vi "Data_Save_MAX.vi"(9 "Data":T1) -> (2 "max":string[](array[string]))   [LabVIEW 2017]
uses:
  Ctrls/Data.ctl
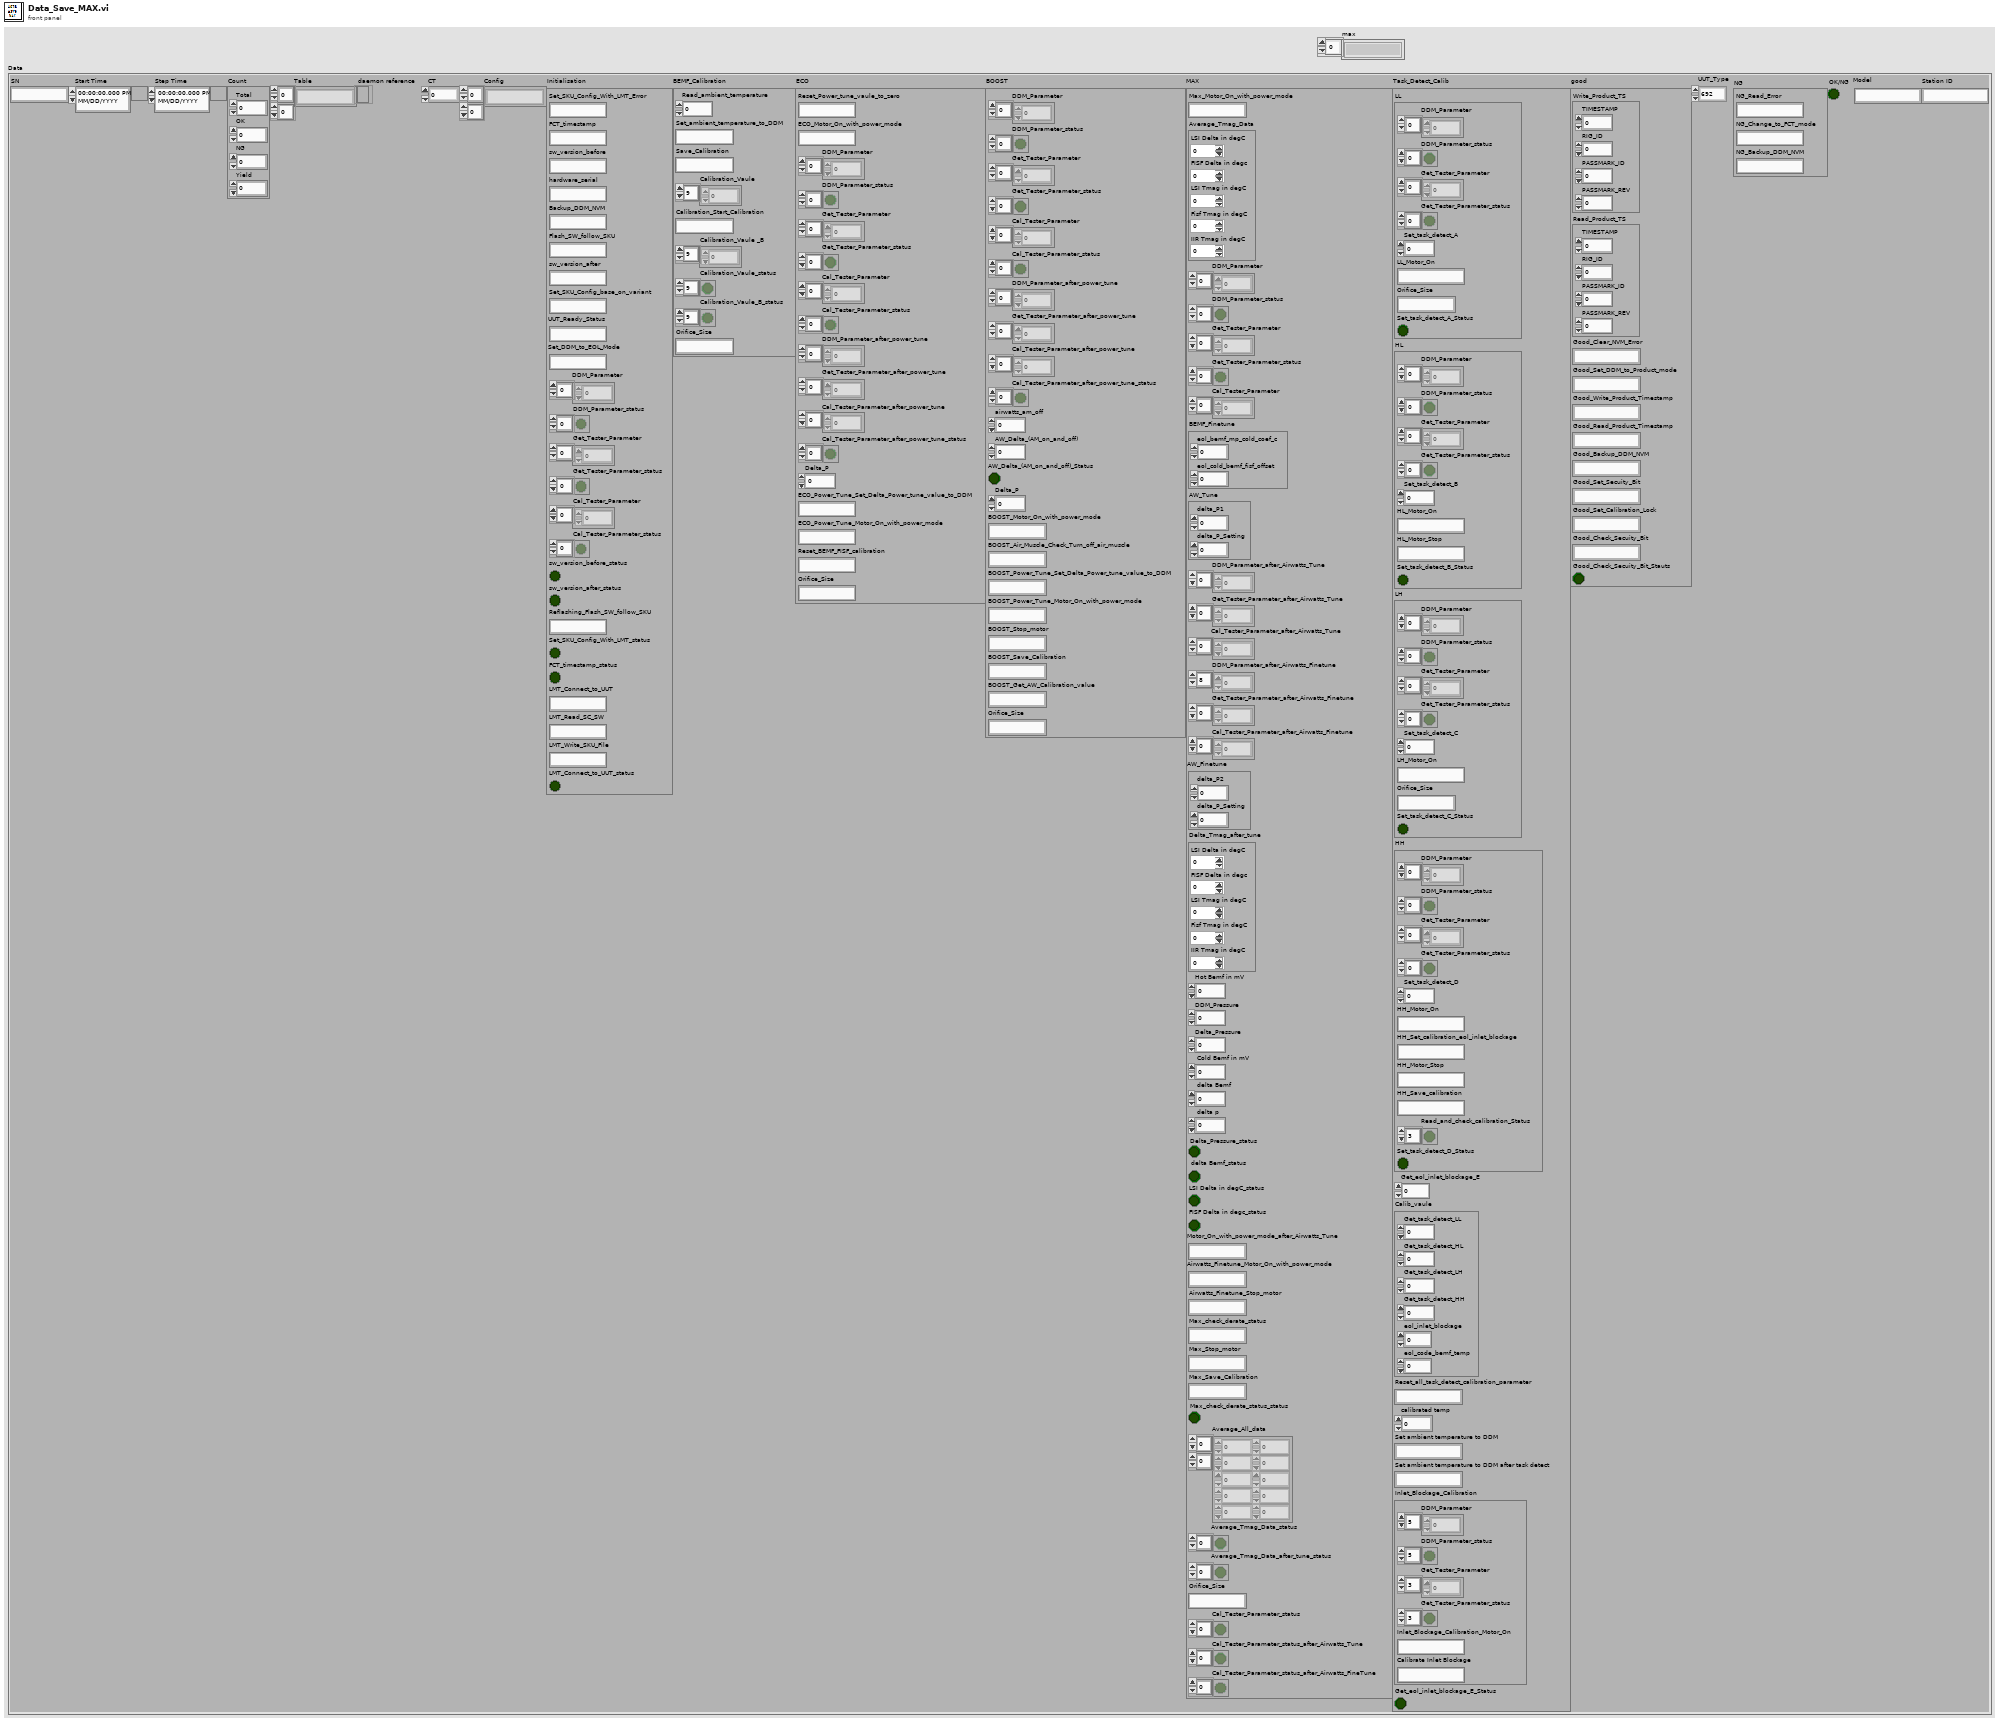
[diagram p1: front panel]
types:
  T1 = typedef "Data.ctl" = cluster{"SN":string, "Start Time":timestamp, "Step Time":timestamp, "Count":cluster{"Total":i32, "OK":i32, "NG":i32, "Yield":dbl}, "Table":string[][], "daemon reference":refnum<k5>, "CT":dbl, "Config":string[][], "Initialisation":cluster{"Set_SKU_Config_With_LMT_Error":string, "FCT_timestamp":string, "sw_version_before":string, "hardware_serial":string, "Backup_DDM_NVM":string, "Flash_SW_follow_SKU":string, "sw_version_after":string, "Set_SKU_Config_base_on_variant":string, "UUT_Ready_Status":string, "Set_DDM_to_EOL_Mode":string, "DDM_Parameter":dbl[], "DDM_Parameter_status":bool[], "Get_Tester_Parameter":dbl[], "Get_Tester_Parameter_status":bool[], "Cal_Tester_Parameter":dbl[], "Cal_Tester_Parameter_status":bool[], "sw_version_before_status":bool, "sw_version_after_status":bool, "Reflashing_Flash_SW_follow_SKU":string, "Set_SKU_Config_With_LMT_status":bool, "FCT_timestamp_status":bool, "LMT_Connect_to_UUT":string, "LMT_Read_SC_SW":string, "LMT_Write_SKU_File":string, "LMT_Connect_to_UUT_status":bool}, "BEMF_Calibration":cluster{"Read_ambient_temperature":dbl, "Set_ambient_temperature_to_DDM":string, "Save_Calibration":string, "Calibration_Vaule":dbl[], "Calibration_Start_Calibration":string, "Calibration_Vaule _B":dbl[], "Calibration_Vaule_status":bool[], "Calibration_Vaule_B_status":bool[], "Orifice_Size":string}, "ECO":cluster{"Reset_Power_tune_vaule_to_zero":string, "ECO_Motor_On_with_power_mode":string, "DDM_Parameter":dbl[], "DDM_Parameter_status":bool[], "Get_Tester_Parameter":dbl[], "Get_Tester_Parameter_status":bool[], "Cal_Tester_Parameter":dbl[], "Cal_Tester_Parameter_status":bool[], "DDM_Parameter_after_power_tune":dbl[], "Get_Tester_Parameter_after_power_tune":dbl[], "Cal_Tester_Parameter_after_power_tune":dbl[], "Cal_Tester_Parameter_after_power_tune_status":bool[], "Delta_P":dbl, "ECO_Power_Tune_Set_Delta_Power_tune_value_to_DDM":string, "ECO_Power_Tune_Motor_On_with_power_mode":string, "Reset_BEMF_FISF_calibration":string, "Orifice_Size":string}, "BOOST":cluster{"DDM_Parameter":dbl[], "DDM_Parameter_status":bool[], "Get_Tester_Parameter":dbl[], "Get_Tester_Parameter_status":bool[], "Cal_Tester_Parameter":dbl[], "Cal_Tester_Parameter_status":bool[], "DDM_Parameter_after_power_tune":dbl[], "Get_Tester_Parameter_after_power_tune":dbl[], "Cal_Tester_Parameter_after_power_tune":dbl[], "Cal_Tester_Parameter_after_power_tune_status":bool[], "airwatts_am_off":dbl, "AW_Delta_(AM_on_and_off)":dbl, "AW_Delta_(AM_on_and_off)_Status":bool, "Delta_P":dbl, "BOOST_Motor_On_with_power_mode":string, "BOOST_Air_Muscle_Check_Turn_off_air_muscle":string, "BOOST_Power_Tune_Set_Delta_Power_tune_value_to_DDM":string, "BOOST_Power_Tune_Motor_On_with_power_mode":string, "BOOST_Stop_motor":string, "BOOST_Save_Calibration":string, "BOOST_Get_AW_Calibration_value":string, "Orifice_Size":string}, "MAX":cluster{"Max_Motor_On_with_power_mode":string, "Average_Tmag_Data":cluster{"LSI Delta in degC":dbl, "FISF Delta in degc":dbl, "LSI Tmag in degC":dbl, "Fisf Tmag in degC":dbl, "IIR Tmag in degC":dbl}, "DDM_Parameter":dbl[], "DDM_Parameter_status":bool[], "Get_Tester_Parameter":dbl[], "Get_Tester_Parameter_status":bool[], "Cal_Tester_Parameter":dbl[], "BEMF_Finetune":cluster{"eol_bemf_mp_cold_coef_c":dbl, "eol_cold_bemf_fisf_offset":dbl}, "AW_Tune":cluster{"delta_P1":dbl, "delta_P_Setting":dbl}, "DDM_Parameter_after_Airwatts_Tune":dbl[], "Get_Tester_Parameter_after_Airwatts_Tune":dbl[], "Cal_Tester_Parameter_after_Airwatts_Tune":dbl[], "DDM_Parameter_after_Airwatts_Finetune":dbl[], "Get_Tester_Parameter_after_Airwatts_Finetune":dbl[], "Cal_Tester_Parameter_after_Airwatts_Finetune":dbl[], "AW_Finetune":cluster{"delta_P2":dbl, "delta_P_Setting":dbl}, "Delta_Tmag_after_tune":cluster{"LSI Delta in degC":dbl, "FISF Delta in degc":dbl, "LSI Tmag in degC":dbl, "Fisf Tmag in degC":dbl, "IIR Tmag in degC":dbl}, "Hot Bemf in mV":dbl, "DDM_Pressure":dbl, "Delta_Pressure":dbl, " Cold Bemf in mV":dbl, " delta Bemf":dbl, " delta p":dbl, "Delta_Pressure_status":bool, " delta Bemf_status":bool, "LSI Delta in degC_status":bool, "FISF Delta in degc_status":bool, "Motor_On_with_power_mode_after_Airwatts_Tune":string, "Airwatts_Finetune_Motor_On_with_power_mode":string, "Airwatts_Finetune_Stop_motor":string, "Max_check_derate_status":string, "Max_Stop_motor":string, "Max_Save_Calibration":string, "Max_check_derate_status_status":bool, "Average_All_data":dbl[][], "Average_Tmag_Data_status":bool[], "Average_Tmag_Data_after_tune_status":bool[], "Orifice_Size":string, "Cal_Tester_Parameter_status":bool[], "Cal_Tester_Parameter_status_after_Airwatts_Tune":bool[], "Cal_Tester_Parameter_status_after_Airwatts_FineTune":bool[]}, "Task_Detect_Calib":cluster{"LL":cluster{"DDM_Parameter":dbl[], "DDM_Parameter_status":bool[], "Get_Tester_Parameter":dbl[], "Get_Tester_Parameter_status":bool[], "Set_task_detect_A":dbl, "LL_Motor_On":string, "Orifice_Size":string, "Set_task_detect_A_Status":bool}, "HL":cluster{"DDM_Parameter":dbl[], "DDM_Parameter_status":bool[], "Get_Tester_Parameter":dbl[], "Get_Tester_Parameter_status":bool[], "Set_task_detect_B":dbl, "HL_Motor_On":string, "HL_Motor_Stop":string, "Set_task_detect_B_Status":bool}, "LH":cluster{"DDM_Parameter":dbl[], "DDM_Parameter_status":bool[], "Get_Tester_Parameter":dbl[], "Get_Tester_Parameter_status":bool[], "Set_task_detect_C":dbl, "LH_Motor_On":string, "Orifice_Size":string, "Set_task_detect_C_Status":bool}, "HH":cluster{"DDM_Parameter":dbl[], "DDM_Parameter_status":bool[], "Get_Tester_Parameter":dbl[], "Get_Tester_Parameter_status":bool[], "Set_task_detect_D":dbl, "HH_Motor_On":string, "HH_Set_calibration_eol_inlet_blockage":string, "HH_Motor_Stop":string, "HH_Save_calibration":string, "Read_and_check_calibration_Status":bool[], "Set_task_detect_D_Status":bool}, "Get_eol_inlet_blockage_E":dbl, "Calib_vaule":cluster{"Get_task_detect_LL":dbl, "Get_task_detect_HL":dbl, "Get_task_detect_LH":dbl, "Get_task_detect_HH":dbl, "eol_inlet_blockage":dbl, "eol_code_bemf_temp":dbl}, "Reset_all_task_detect_calibration_parameter":string, "calibrated temp":dbl, "Set ambient temperature to DDM":string, "Set ambient temperature to DDM after task detect":string, "Inlet_Blockage_Calibration":cluster{"DDM_Parameter":dbl[], "DDM_Parameter_status":bool[], "Get_Tester_Parameter":dbl[], "Get_Tester_Parameter_status":bool[], "Inlet_Blockage_Calibration_Motor_On":string, "Calibrate Inlet Blockage":string}, "Get_eol_inlet_blockage_E_Status":bool}, "good":cluster{"Write_Product_TS":cluster{"TIMESTAMP":i64, "RIG_ID":i64, "PASSMARK_ID":i64, "PASSMARK_REV":i64}, "Read_Product_TS":cluster{"TIMESTAMP":i64, "RIG_ID":i64, "PASSMARK_ID":i64, "PASSMARK_REV":i64}, "Good_Clear_NVM_Error":string, "Good_Set_DDM_to_Product_mode":string, "Good_Write_Product_Timestamp":string, "Good_Read_Product_Timestamp":string, "Good_Backup_DDM_NVM":string, "Good_Set_Secuity_Bit":string, "Good_Set_Calibration_Lock":string, "Good_Check_Secuity_Bit":string, "Good_Check_Secuity_Bit_Stauts":bool}, "UUT_Type":enum16{"692", "692B", "692D"}, "NG":cluster{"NG_Read_Error":string, "NG_Change_to_FCT_mode":string, "NG_Backup_DDM_NVM":string}, "OK/NG":bool, "Model":string, "Station ID":string}
  T2 = cluster{"LSI Delta in degC":dbl, "FISF Delta in degc":dbl, "LSI Tmag in degC":dbl, "Fisf Tmag in degC":dbl, "IIR Tmag in degC":dbl}
  T3 = typedef "HD Config.ctl" = cluster{" PC":cluster{"PC Address":u8[], "PC Port":i32}, "FCO":cluster{"COM":refnum<visa-resource-name>, "Baudrate":u32}, "DC Power ":cluster{"COM":refnum<visa-resource-name>, "Baudrate":u32}, "PW3336":cluster{"COM":refnum<visa-resource-name>, "Baudrate":u32}, "Lefoo":cluster{"COM":refnum<visa-resource-name>, "Baudrate":u32}, "AI Model":cluster{"COM":refnum<visa-resource-name>, "Baudrate":u32}, "DIPC":cluster{"COM":refnum<visa-resource-name>}, "Daemon":cluster{"IP Address":string, "Port":u16, "Retry":u16}, "Motor":cluster{"COM":refnum<visa-resource-name>, "Baudrate":u32}, "G1":bool, "Fail_resume_mode":bool, "Skip DDM Speed&Pressure Passmark":bool}
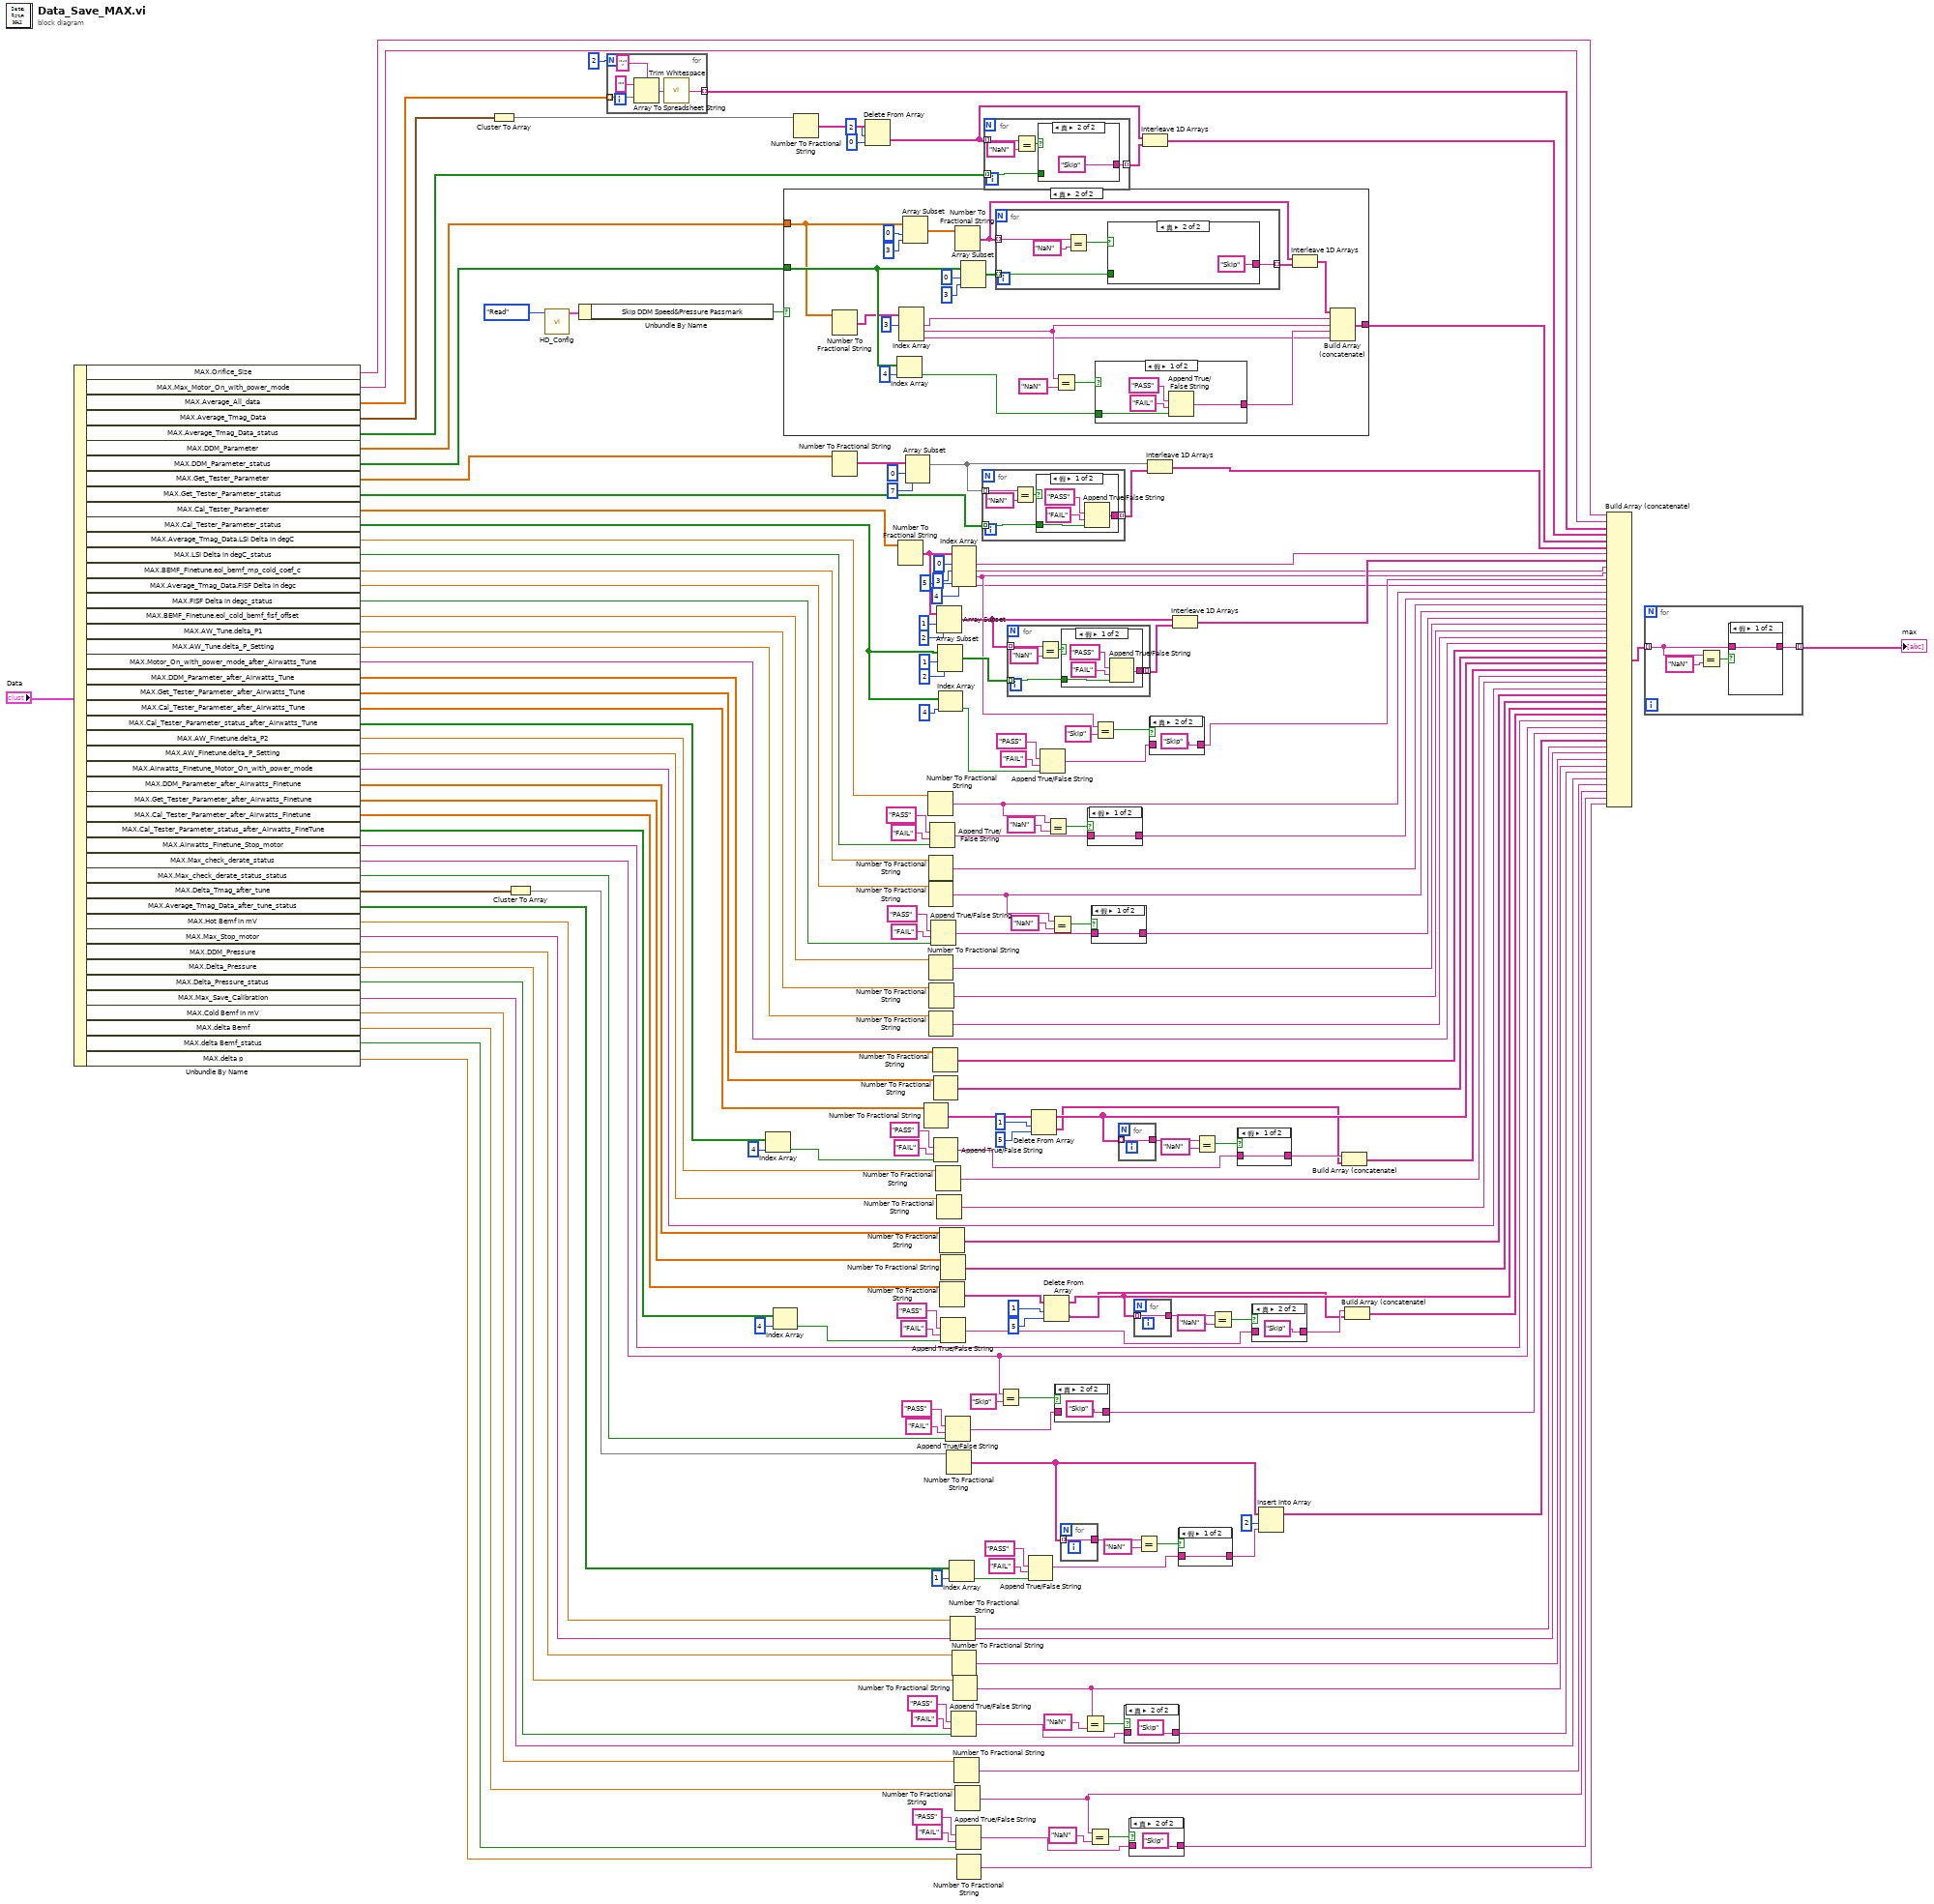
[diagram p0: block diagram]
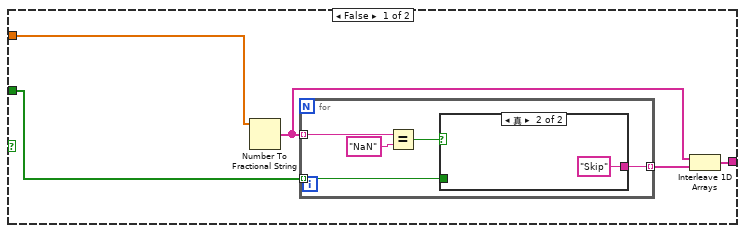
[diagram p2: hidden frame]
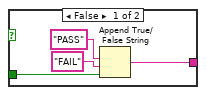
[diagram p3: hidden frame]
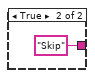
[diagram p4: hidden frame]
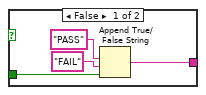
[diagram p5: hidden frame]
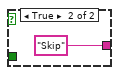
[diagram p7: hidden frame]
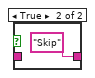
[diagram p8: hidden frame]
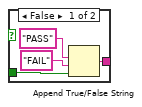
[diagram p9: hidden frame]
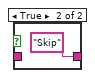
[diagram p14: hidden frame]
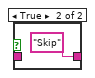
[diagram p15: hidden frame]
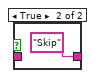
[diagram p16: hidden frame]
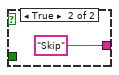
[diagram p17: hidden frame]
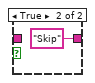
[diagram p18: hidden frame]
diagram:
  n1 = Unbundle By Name("Data") -> ("MAX.Orifice_Size"=w56:string, "MAX.Max_Motor_On_with_power_mode"=w57:string, "MAX.Average_All_data"=w80:dbl[][], "MAX.Average_Tmag_Data"=w177:T2, "MAX.Average_Tmag_Data_status"=w75:bool[], "MAX.DDM_Parameter"=w24:dbl[], "MAX.DDM_Parameter_status"=w23:bool[], "MAX.Get_Tester_Parameter"=w175:dbl[], "MAX.Get_Tester_Parameter_status"=w126:bool[], "MAX.Cal_Tester_Parameter"=w174:dbl[], "MAX.Cal_Tester_Parameter_status"=w47:bool[], "MAX.Average_Tmag_Data.LSI Delta in degC"=w172:dbl, "MAX.LSI Delta in degC_status"=w171:bool, "MAX.BEMF_Finetune.eol_bemf_mp_cold_coef_c"=w170:dbl, "MAX.Average_Tmag_Data.FISF Delta in degc"=w169:dbl, "MAX.FISF Delta in degc_status"=w168:bool, "MAX.BEMF_Finetune.eol_cold_bemf_fisf_offset"=w167:dbl, "MAX.AW_Tune.delta_P1"=w166:dbl, "MAX.AW_Tune.delta_P_Setting"=w165:dbl, "MAX.Motor_On_with_power_mode_after_Airwatts_Tune"=w160:string, "MAX.DDM_Parameter_after_Airwatts_Tune"=w159:dbl[], "MAX.Get_Tester_Parameter_after_Airwatts_Tune"=w158:dbl[], "MAX.Cal_Tester_Parameter_after_Airwatts_Tune"=w14:dbl[], "MAX.Cal_Tester_Parameter_status_after_Airwatts_Tune"=w155:bool[], "MAX.AW_Finetune.delta_P2"=w154:dbl, "MAX.AW_Finetune.delta_P_Setting"=w153:dbl, "MAX.Airwatts_Finetune_Motor_On_with_power_mode"=w150:string, "MAX.DDM_Parameter_after_Airwatts_Finetune"=w147:dbl[], "MAX.Get_Tester_Parameter_after_Airwatts_Finetune"=w146:dbl[], "MAX.Cal_Tester_Parameter_after_Airwatts_Finetune"=w145:dbl[], "MAX.Cal_Tester_Parameter_status_after_Airwatts_FineTune"=w144:bool[], "MAX.Airwatts_Finetune_Stop_motor"=w141:string, "MAX.Max_check_derate_status"=w84:string, "MAX.Max_check_derate_status_status"=w86:bool, "MAX.Delta_Tmag_after_tune"=w176:T2, "MAX.Average_Tmag_Data_after_tune_status"=w71:bool[], "MAX.Hot Bemf in mV"=w139:dbl, "MAX.Max_Stop_motor"=w137:string, "MAX.DDM_Pressure"=w136:dbl, "MAX.Delta_Pressure"=w89:dbl, "MAX.Delta_Pressure_status"=w92:bool, "MAX.Max_Save_Calibration"=w134:string, "MAX.Cold Bemf in mV"=w133:dbl, "MAX.delta Bemf"=w132:dbl, "MAX.delta Bemf_status"=w100:bool, "MAX.delta p"=w131:dbl)
  n2 = Cluster To Array(cluster=w177) -> (array=w173:dbl[])
  n3 = Cluster To Array(cluster=w176) -> (array=w140:dbl[])
  n4 = call "HD_Config.vi"("Step"=enum16{"Initial", "Write", "Read"}."Read") -> ("HD Config out"=w26:T3)  [unwired: 9 in, 1 out]
  n5 = Unbundle By Name(w26) -> ("Skip DDM Speed&Pressure Passmark"=w25:bool)
  n6 = for {
    N: 2 -> [_]
    tunnel: w80 -> [w189] mode=indexing
    tunnel: [w185] -> w79 mode=indexing
    n7 = Array To Spreadsheet String(delimiter (Tab)=";", array=w189, 3:"" ("format string")) -> (spreadsheet string=w186:string)
    n8 = call <vilib>:"Trim Whitespace.vi"("string"=w186) -> ("trimmed string"=w185:string)  [unwired: 1 in]
  }
  n9 = Index Array(array=w155, index=4) -> (element=w34:bool)
  n10 = Index Array(array=w144, index=4) -> (element=w32:bool)
  n11 = case shown="真" w25 {
    tunnel: w23 -> [w190 w216]
    tunnel: w24 -> [w191 w213]
    tunnel: [w192 w205] -> w22
    frame False {
      n12 = Number To Fractional String(number=w191) -> (F-format string=w193:string[])  [unwired: 3 in]
      n13 = for {
        tunnel: w190 -> [w199] mode=indexing
        tunnel: [w198] -> w194 mode=indexing
        tunnel: w193 -> [w196] mode=indexing
        n14 = Equal?(x=w196, y="NaN" ("x")) -> (x = y?=w195:bool)
        n15 = case shown="真" w195 {
          tunnel: w199 -> [w203 _]
          tunnel: [w201 "Skip" ("x")] -> w198
          frame False {
            n16 = Append True/False String(1:w203, 2:"FAIL" ("字符串(\"\")"), 3:"PASS" ("真字符串")) -> (0:w201:string)  [unwired: 1 in]
          }
          frame True {
          }
        }
      }
      n17 = Interleave 1D Arrays(w193, w194) -> (w192:string[])
    }
    frame True {
      n18 = Number To Fractional String(number=w213) -> (F-format string=w212:string[])  [unwired: 3 in]
      n19 = Index Array(array=w216, index=4 ("索引")) -> (element=w211:bool)
      n20 = Index Array(array=w212, index #1=3 ("索引")) -> (element #1=w210:string, element #2=w208:string, element #3=w207:string)  [unwired: 2 in]
      n21 = Array Subset(array=w213, index=0 ("索引"), length=3 ("长度")) -> (w224:dbl[])
      n22 = Number To Fractional String(number=w224) -> (F-format string=w219:string[])  [unwired: 3 in]
      n23 = Array Subset(array=w216, index=0 ("索引"), length=3 ("长度")) -> (w225:bool[])
      n24 = for {
        tunnel: w225 -> [w236] mode=indexing
        tunnel: [w235] -> w226 mode=indexing
        tunnel: w219 -> [w233] mode=indexing
        n25 = Equal?(x=w233, y="NaN" ("x")) -> (x = y?=w232:bool)
        n26 = case shown="真" w232 {
          tunnel: w236 -> [w240 _]
          tunnel: [w238 "Skip" ("x")] -> w235
          frame False {
            n27 = Append True/False String(1:w240, 2:"FAIL" ("字符串(\"\")"), 3:"PASS" ("真字符串")) -> (0:w238:string)  [unwired: 1 in]
          }
          frame True {
          }
        }
      }
      n28 = Equal?(x=w208, y="NaN" ("x")) -> (x = y?=w215:bool)
      n29 = case shown="假" w215 {
        tunnel: w211 -> [w230 _]
        tunnel: [w228 "Skip" ("x")] -> w209
        frame False {
          n30 = Append True/False String(1:w230, 2:"FAIL" ("字符串(\"\")"), 3:"PASS" ("真字符串")) -> (0:w228:string)  [unwired: 1 in]
        }
        frame True {
        }
      }
      n31 = Interleave 1D Arrays(w219, w226) -> (w206:string[])
      n32 = Build Array (concatenate)(w206, w210, w208, w209, w207) -> (w205:string[])
    }
  }
  n33 = Number To Fractional String(number=w173) -> (F-format string=w78:string[])  [unwired: 3 in]
  n34 = Number To Fractional String(number=w175) -> (F-format string=w18:string[])  [unwired: 3 in]
  n35 = Delete From Array(array=w78, length=2, index=0) -> (deleted portion=w74:string[])  [unwired: 1 out]
  n36 = Number To Fractional String(number=w174) -> (F-format string=w55:string[])  [unwired: 3 in]
  n37 = Array Subset(array=w18, index=0 ("索引"), length=7 ("长度")) -> (w21:string[])
  n38 = Number To Fractional String(number=w14) -> (F-format string=w10:string[])  [unwired: 3 in]
  n39 = Number To Fractional String(number=w172) -> (F-format string=w122:string)  [unwired: 3 in]
  n40 = Number To Fractional String(number=w170) -> (F-format string=w164:string)  [unwired: 3 in]
  n41 = Number To Fractional String(number=w169) -> (F-format string=w116:string)  [unwired: 3 in]
  n42 = Number To Fractional String(number=w167) -> (F-format string=w163:string)  [unwired: 3 in]
  n43 = Number To Fractional String(number=w165) -> (F-format string=w161:string)  [unwired: 3 in]
  n44 = Number To Fractional String(number=w166) -> (F-format string=w162:string)  [unwired: 3 in]
  n45 = Append True/False String(1:w171, 2:"FAIL" ("字符串(\"\")"), 3:"PASS" ("真字符串")) -> (0:w121:string)  [unwired: 1 in]
  n46 = Append True/False String(1:w168, 2:"FAIL" ("字符串(\"\")"), 3:"PASS" ("真字符串")) -> (0:w117:string)  [unwired: 1 in]
  n47 = Number To Fractional String(number=w159) -> (F-format string=w157:string[])  [unwired: 3 in]
  n48 = Number To Fractional String(number=w158) -> (F-format string=w156:string[])  [unwired: 3 in]
  n49 = Append True/False String(1:w34, 2:"FAIL" ("字符串(\"\")"), 3:"PASS" ("真字符串")) -> (0:w111:string)  [unwired: 1 in]
  n50 = Number To Fractional String(number=w154) -> (F-format string=w152:string)  [unwired: 3 in]
  n51 = Array Subset(array=w55, index=1, length=2) -> (w45:string[])
  n52 = Number To Fractional String(number=w153) -> (F-format string=w151:string)  [unwired: 3 in]
  n53 = Array Subset(array=w47, index=1, length=2) -> (w44:bool[])
  n54 = Index Array(array=w47, index=4) -> (element=w38:bool)
  n55 = Number To Fractional String(number=w147) -> (F-format string=w143:string[])  [unwired: 3 in]
  n56 = Number To Fractional String(number=w145) -> (F-format string=w5:string[])  [unwired: 3 in]
  n57 = Number To Fractional String(number=w146) -> (F-format string=w142:string[])  [unwired: 3 in]
  n58 = Append True/False String(1:w32, 2:"FAIL" ("字符串(\"\")"), 3:"PASS" ("真字符串")) -> (0:w106:string)  [unwired: 1 in]
  n59 = Append True/False String(1:w86, 2:"FAIL" ("字符串(\"\")"), 3:"PASS" ("真字符串")) -> (0:w82:string)  [unwired: 1 in]
  n60 = Number To Fractional String(number=w140) -> (F-format string=w61:string[])  [unwired: 3 in]
  n61 = Index Array(array=w71, index=1) -> (element=w66:bool)
  n62 = Number To Fractional String(number=w139) -> (F-format string=w138:string)  [unwired: 3 in]
  n63 = Append True/False String(1:w92, 2:"FAIL" ("字符串(\"\")"), 3:"PASS" ("真字符串")) -> (0:w97:string)  [unwired: 1 in]
  n64 = Index Array(array=w55, index #1=0 ("index"), index #2=3 ("index"), index #3=4 ("index"), index #4=5 ("索引")) -> (element #1=w35:string, element #2=w29:string, element #3=w28:string, element #4=w15:string)
  n65 = Number To Fractional String(number=w136) -> (F-format string=w135:string)  [unwired: 3 in]
  n66 = Number To Fractional String(number=w89) -> (F-format string=w91:string)  [unwired: 3 in]
  n67 = Number To Fractional String(number=w133) -> (F-format string=w130:string)  [unwired: 3 in]
  n68 = Number To Fractional String(number=w132) -> (F-format string=w101:string)  [unwired: 3 in]
  n69 = Append True/False String(1:w100, 2:"FAIL" ("字符串(\"\")"), 3:"PASS" ("真字符串")) -> (0:w99:string)  [unwired: 1 in]
  n70 = Number To Fractional String(number=w131) -> (F-format string=w129:string)  [unwired: 3 in]
  n71 = for {
    tunnel: w126 -> [w246] mode=indexing
    tunnel: [w245] -> w125 mode=indexing
    tunnel: w21 -> [w243] mode=indexing
    n72 = Equal?(x=w243, y="NaN" ("x")) -> (x = y?=w242:bool)
    n73 = case shown="假" w242 {
      tunnel: w246 -> [w250 _]
      tunnel: [w248 "Skip" ("x")] -> w245
      frame False {
        n74 = Append True/False String(1:w250, 2:"FAIL" ("字符串(\"\")"), 3:"PASS" ("真字符串")) -> (0:w248:string)  [unwired: 1 in]
      }
      frame True {
      }
    }
  }
  n75 = for {
    tunnel: w75 -> [w256] mode=indexing
    tunnel: [w255] -> w73 mode=indexing
    tunnel: w74 -> [w253] mode=indexing
    n76 = Equal?(x=w253, y="NaN" ("x")) -> (x = y?=w252:bool)
    n77 = case shown="真" w252 {
      tunnel: w256 -> [w260 _]
      tunnel: [w258 "Skip" ("x")] -> w255
      frame False {
        n78 = Append True/False String(1:w260, 2:"FAIL" ("字符串(\"\")"), 3:"PASS" ("真字符串")) -> (0:w258:string)  [unwired: 1 in]
      }
      frame True {
      }
    }
  }
  n79 = Equal?(x=w84, y="Skip" ("x")) -> (x = y?=w83:bool)
  n80 = for {
    tunnel: w44 -> [w266] mode=indexing
    tunnel: [w265] -> w46 mode=indexing
    tunnel: w45 -> [w263] mode=indexing
    n81 = Equal?(x=w263, y="NaN" ("x")) -> (x = y?=w262:bool)
    n82 = case shown="假" w262 {
      tunnel: w266 -> [w270 _]
      tunnel: [w268 "Skip" ("x")] -> w265
      frame False {
        n83 = Append True/False String(1:w270, 2:"FAIL" ("字符串(\"\")"), 3:"PASS" ("真字符串")) -> (0:w268:string)  [unwired: 1 in]
      }
      frame True {
      }
    }
  }
  n84 = Append True/False String(1:w66, 2:"FAIL" ("字符串(\"\")"), 3:"PASS" ("真字符串")) -> (0:w62:string)  [unwired: 1 in]
  n85 = Delete From Array(array=w10, length=1 ("长度"), index=5 ("索引")) -> (deleted portion=w8:string[], array with subset deleted=w11:string[])
  n86 = Append True/False String(1:w38, 2:"FAIL" ("字符串(\"\")"), 3:"PASS" ("真字符串")) -> (0:w43:string)  [unwired: 1 in]
  n87 = Delete From Array(array=w5, length=1 ("长度"), index=5 ("索引")) -> (deleted portion=w1:string[], array with subset deleted=w4:string[])
  n88 = Equal?(x=w122, y="NaN" ("x")) -> (x = y?=w123:bool)
  n89 = Equal?(x=w116, y="NaN" ("x")) -> (x = y?=w119:bool)
  n90 = case shown="真" w83 {
    tunnel: [w272 "Skip" ("x")] -> w81
    tunnel: w82 -> [w272 _]
    frame False {
    }
    frame True {
    }
  }
  n91 = for {
    tunnel: w61 -> [w274] mode=indexing
    tunnel: [w274] -> w63
  }
  n92 = Equal?(x=w91, y="NaN" ("x")) -> (x = y?=w93:bool)
  n93 = case shown="假" w123 {
    tunnel: [w275 "Skip" ("x")] -> w120
    tunnel: w121 -> [w275 _]
    frame False {
    }
    frame True {
    }
  }
  n94 = Equal?(x=w101, y="NaN" ("x")) -> (x = y?=w105:bool)
  n95 = case shown="假" w119 {
    tunnel: [w277 "Skip" ("x")] -> w115
    tunnel: w117 -> [w277 _]
    frame False {
    }
    frame True {
    }
  }
  n96 = Equal?(x=w28, y="Skip" ("x")) -> (x = y?=w42:bool)
  n97 = for {
    tunnel: w11 -> [w279] mode=indexing
    tunnel: [w279] -> w114
  }
  n98 = case shown="真" w93 {
    tunnel: [w280 "Skip" ("x")] -> w90
    tunnel: w97 -> [w280 _]
    frame False {
    }
    frame True {
    }
  }
  n99 = case shown="真" w105 {
    tunnel: [w282 "Skip" ("x")] -> w98
    tunnel: w99 -> [w282 _]
    frame False {
    }
    frame True {
    }
  }
  n100 = for {
    tunnel: w4 -> [w284] mode=indexing
    tunnel: [w284] -> w107
  }
  n101 = Equal?(x=w63, y="NaN" ("x")) -> (x = y?=w65:bool)
  n102 = Interleave 1D Arrays(w74, w73) -> (w72:string[])
  n103 = Interleave 1D Arrays(w21, w125) -> (w17:string[])
  n104 = case shown="真" w42 {
    tunnel: [w285 "Skip" ("x")] -> w37
    tunnel: w43 -> [w285 _]
    frame False {
    }
    frame True {
    }
  }
  n105 = Interleave 1D Arrays(w45, w46) -> (w36:string[])
  n106 = case shown="假" w65 {
    tunnel: [w287 "Skip" ("x")] -> w60
    tunnel: w62 -> [w287 _]
    frame False {
    }
    frame True {
    }
  }
  n107 = Equal?(x=w114, y="NaN" ("x")) -> (x = y?=w112:bool)
  n108 = Equal?(x=w107, y="NaN" ("x")) -> (x = y?=w109:bool)
  n109 = case shown="假" w112 {
    tunnel: [w289 "Skip" ("x")] -> w110
    tunnel: w111 -> [w289 _]
    frame False {
    }
    frame True {
    }
  }
  n110 = case shown="真" w109 {
    tunnel: [w291 "Skip" ("x")] -> w3
    tunnel: w106 -> [w291 _]
    frame False {
    }
    frame True {
    }
  }
  n111 = Insert Into Array(array=w61, index=2, new element=w60) -> (w59:string[])
  n112 = Build Array (concatenate)(w110, w8) -> (w9:string[])
  n113 = Build Array (concatenate)(w3, w1) -> (w2:string[])
  n114 = Build Array (concatenate)(w56, w57, w79, w72, w22, w17, w35, w36, w29, w28, w37, w15, w122, w120, w164, w116, w115, w163, w162, w161, w160, w157, w156, w11, w9, w152, w151, w150, w143, w142, w4, w2, w141, w84, w81, w59, w138, w137, w135, w91, w90, w134, w130, w101, w98, w129) -> (w128:string[])
  n115 = for {
    tunnel: [w296] -> w127 mode=indexing
    tunnel: w128 -> [w293] mode=indexing
    n116 = Equal?(x=w293, y="NaN" ("x")) -> (x = y?=w294:bool)
    n117 = case shown="假" w294 {
      tunnel: [w297 "Skip" ("x")] -> w296
      tunnel: w293 -> [w297 _]
      frame False {
      }
      frame True {
      }
    }
  }
  "max" <- w127
